vi "LoadPluginRequest.vi"(8 "error in (no error)":errorcluster, 10 "PathToPlugin":path, 11 "ModuleID":i32=-1) -> (0 "error out":errorcluster)   [LabVIEW 2017, in "NetworkImpairmentModule.lvlib"]
uses:
  NetworkImpairmentModule.lvlib
  clEventType.ctl
  <vilib>/Utility/error.llb/Error Cluster From Error Code.vi
  <vilib>/ErrorRing/Error Ring.xnode
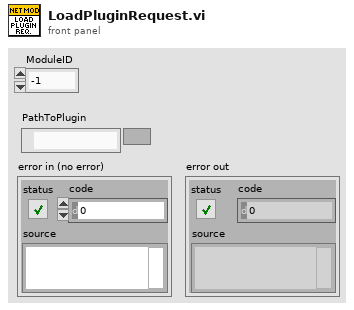
[diagram p1: front panel]
types:
  T1 = typedef "NetworkImpairmentModule.lvlib/clRequestEvents.ctl" = cluster{"StopRequest":refnum<user-event>, "WriteTimeArrayRequest":refnum<user-event>, "WriteNetImpParamsRequest":refnum<user-event>, "ReadNetImpParamsRequest":refnum<user-event>, "WriteLossThresholdRequest":refnum<user-event>, "ReadLossThresholdRequest":refnum<user-event>, "GetNetworkTimeRequest":refnum<user-event>, "GetPktLossRequest":refnum<user-event>, "LoadPluginRequest":refnum<user-event>, "ReadPathToPluginRequest":refnum<user-event>, "ShowPanel":refnum<user-event>}
  T2 = typedef "NetworkImpairmentModule.lvlib/clEventType.ctl" = cluster{"ModuleID":i32, "Data":variant}
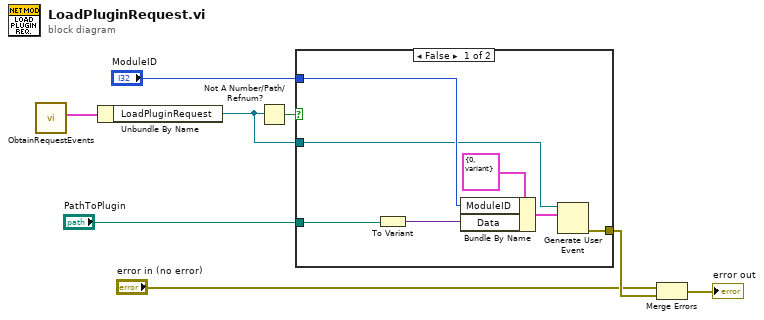
[diagram p0: block diagram]
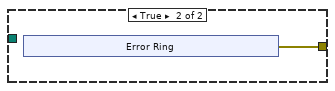
[diagram p2: hidden frame]
diagram:
  n1 = call "ObtainRequestEvents.vi"() -> ("clRequestEvents"=w8:T1)  [unwired: 10 in, 1 out]
  n2 = Unbundle By Name(w8) -> ("LoadPluginRequest"=w6:refnum<user-event>)
  n3 = Not A Number/Path/Refnum?(number/path/refnum=w6) -> (NaN/Path/Refnum?=w7:bool)
  n4 = case shown="False" w7 {
    tunnel: w6 -> [w13 _]
    tunnel: "ModuleID" -> [w14 _]
    tunnel: "PathToPlugin" -> [w10 _]
    tunnel: [w11 w16] -> w3
    frame False {
      n5 = To Variant(anything=w10) -> (Variant=w9:variant)
      n6 = Bundle By Name(cluster=T2 {"ModuleID"=0, "Data"=variant} ("clEventType"), "ModuleID"=w14, "Data"=w9) -> (w12:T2)
      n7 = Generate User Event(user event=w13, event data cluster=w12) -> (error out=w11:errorcluster)  [unwired: 2 in, 1 out]
    }
    frame True {
      n8 = xnode "Error Ring"() -> ("error out"=w16:errorcluster)
    }
  }
  n9 = Merge Errors("error in (no error)", w3) -> (→"error out":errorcluster)
